vi "NF87XX.destructor.vi"(0 "i ref in":refnum<vi>, 5 "error in(no error)":errorcluster) -> (19 "error out":errorcluster)   [LabVIEW 2014, in "NF87XX.lvlib"]
doc: "This is the destructor of a class.\n\nLicense Agreement for this software:\n\nCopyright (C)\nGesellschaft für Schwerionenforschung, GSI\nPlanckstr. 1\n64291 Darmstadt\nGermany\n\nContact: D.Beck@gsi.de \n\nThis program is free software; you can redistribute it and/or modify it under the terms of the \nGNU General Public License as published by the Free Software Foundation; either version 2 of \nthe license, or (at your option) any later version.\n\nThis program is distributed in the hope that it will be useful, but WITHOUT ANY WARRANTY; \nwithout even the implied warranty of MERCHANTABILITY or FITNESS FOR A PARTICULAR PURPOSE. See the GNU General License for more details (http://www.gnu.org).\n\nGesellschaft für Schwerionenforschung, GSI\nPlanckstr. 1, 64291 Darmstadt, Germany\nFor all questions and ideas contact: M.Richter@gsi.de, H.Brand@gsi.de or D.Beck@gsi.de.\nLast update: 16-JUN-2004"
uses:
  NF87XX.lvlib
  CSCore/BaseProcess/BaseProcess.lvlib
  lib.lib/DimLVEvent/LVDimInterface/LVDimInterface.lvlib
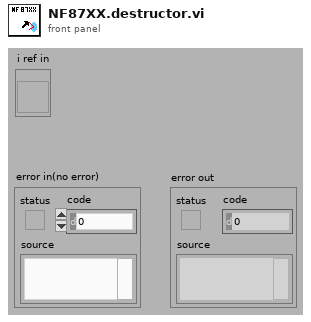
[diagram p1: front panel]
types:
  T1 = enum16{"User....", "DEF", "DIAG", "INI", "LOCK", "UNLOCK", "MAP", "SAV", "VER", "ACC", "CHL", "FOR", "GO", "HAL", "MOF", "MON", "MPV", "POS", "REL", "REV", "STA", "STO", "TYP", "VEL", "ABS", "SER", "NOS", "DRT", "FLI", "RLI", "FIN", "RIN", "AIN", "IN", "JOF", "JON", "OUT", "RES FINE", "RES COARSE", "02 (HEX)", "PWM", "CNT", "TMR", "HOSTNAME", "IPADDR", "IPMODE", "NETMASK", "GATEWAY", "DNSSRVR", "PASSWD", "ECHO", "MACADDR"}
  T2 = enum16{"SetAttribute", "GetAttribute", "CreateAttribute", "DestroyAttribute", "DestroyAllAtributes"}
  T3 = typedef "NF87XX.lvlib/NF87XX.i attribute.ctl" = cluster{"Con Settings":T4, "Drivers":T5[], "Status":cluster{"Service ID":i32, "Status":T8}, "Joystick available":bool, "VISA Resource":string}
  T4 = typedef "NewFocusPico - Driver np.lvlib/VISA & TCPIP Control.ctl" = cluster{"VISA or TCP/IP":bool, "Init Connection":bool, "Close Connection":bool, "Resource Name":refnum<visa-resource-name>, "hostname":string, "connection ID":refnum<k5>}
  T5 = typedef "NF87XX.lvlib/NF87XX.driver Settings.ctl" = cluster{"Name":string, "Driver Type":T6, "Pico Parameter type":T7, "Acceleration [Steps/s²]":cluster{"Motor 0":dbl, "Motor 1":dbl, "Motor 2":dbl}, "Start Velocity [Steps/s]":cluster{"Motor 0":dbl, "Motor 1":dbl, "Motor 2":dbl}, "Velocity [Steps/s]":cluster{"Motor 0":dbl, "Motor 1":dbl, "Motor 2":dbl}, "axis channel":i32, "Position":i32, "Position Service ID":i32}
  T6 = typedef "NF87XX.lvlib/NF87XX.driver Type.ctl" = enum16{"not defined", "3-ch open loop drv", "1-ch closed loop drv"}
  T7 = typedef "NewFocusPico - Driver np.lvlib/Pico Parameters.ctl" = cluster{"Pico Type":enum16{"Open-Loop Pico", "Close-Loop Pico", "Pico Ultra"}, "Acceleration (steps/sec^2)":string, "Velocity ( Hz)":string, "Driver":string, "Motor":string, "Channel":string, "Process Step":string}
  T8 = typedef "PH_StatusHandler.lvlib/PH_StatusHandler.Status.ctl" = i16
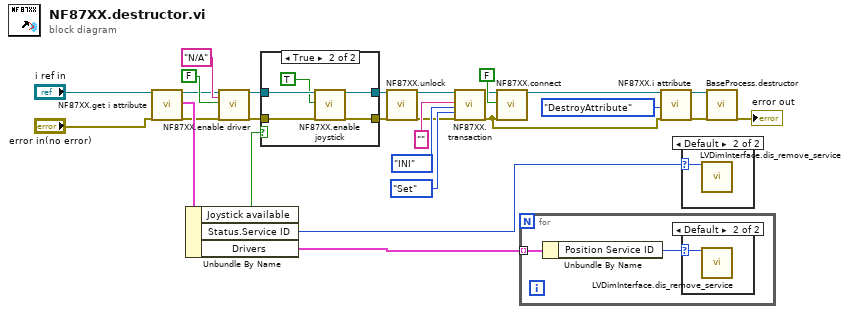
[diagram p0: block diagram]
diagram:
  n1 = call "NF87XX.get i attribute.vi"("i ref in"="i ref in", "error in (no error)"="error in(no error)") -> ("i ref out"=w4:refnum<vi>, "i attribute"=w16:T3, "error out"=w2:errorcluster)  [unwired: 15 in]
  n2 = Unbundle By Name(w16) -> ("Joystick available"=w1:bool, "Status.Service ID"=w14:i32, "Drivers"=w15:T5[])
  n3 = call "NF87XX.enable driver.vi"("i ref in"=w4, "System"="N/A", "Enable Driver"=FALSE, "error in (no error)"=w2) -> ("i ref out"=w11:refnum<vi>, "error out"=w9:errorcluster)  [unwired: 14 in]
  n4 = case shown="True" w1 {
    tunnel: w11 -> [w29 w34]
    tunnel: [w29 w33] -> w10
    tunnel: w9 -> [w28 w32]
    tunnel: [w28 w31] -> w8
    frame False {
    }
    frame True {
      n5 = call "NF87XX.enable joystick.vi"("i ref in"=w34, "Enable Joystick"=TRUE, "error in (no error)"=w32) -> ("i ref out"=w33:refnum<vi>, "error out"=w31:errorcluster)  [unwired: 15 in]
    }
  }
  n6 = call "NF87XX.unlock.vi"("i ref in"=w10, "error in (no error)"=w8) -> ("i ref out"=w17:refnum<vi>, "error out"=w18:errorcluster)  [unwired: 16 in]
  n7 = call "NF87XX.transaction.vi"("i ref in"=w17, "User Cmd/Numeric Argu"="", "MCL Cmd"=T1."INI", "Query/Set"=enum16{"Query", "Set"}."Set", "error in (no error)"=w18) -> ("i ref out"=w7:refnum<vi>, "error out"=w6:errorcluster)  [unwired: 12 in, 1 out]
  n8 = call "NF87XX.connect.vi"("i ref in"=w7, "Connect?"=FALSE ("Enable Driver"), "error in (no error)"=w6) -> ("i ref out"=w23:refnum<vi>)  [unwired: 15 in, 1 out]
  n9 = for {
    tunnel: w15 -> [w36] mode=indexing
    n10 = Unbundle By Name(w36) -> ("Position Service ID"=w35:i32)
    n11 = case shown="Default" w35 {
      selector: w35 -> [_ w37]
      frame -1 {
      }
      frame Default {
        n12 = call "LVDimInterface.dis_remove_service.vi"("my_serviceID"=w37) -> ()  [unwired: 18 in, 1 out]
      }
    }
  }
  n13 = call "NF87XX.i attribute.vi"("VI Refnum"=w23, "Action"=T2."DestroyAttribute", "error in (no error)"=w6) -> ("VI Refnum out"=w26:refnum<vi>, "error out"=w25:errorcluster)  [unwired: 14 in, 1 out]
  n14 = case shown="Default" w14 {
    selector: w14 -> [_ w38]
    frame -1 {
    }
    frame Default {
      n15 = call "LVDimInterface.dis_remove_service.vi"("my_serviceID"=w38) -> ()  [unwired: 18 in, 1 out]
    }
  }
  n16 = call "BaseProcess.destructor.vi"("i ref in"=w26, "error in (no error)"=w25) -> ("error out"=→"error out":errorcluster)  [unwired: 17 in]
